vi "0.初始化饼状图.vi"(8 "error in":errorcluster) -> (0 "error out":errorcluster, 3 "Module ID out":i32)   [LabVIEW 2020, in "PichartInterface.lvlib"]
uses:
  PichartInterface.lvlib
  <vilib>/DD/DDToolsVIPM/PieChartInterface/PieChart.lvlibp
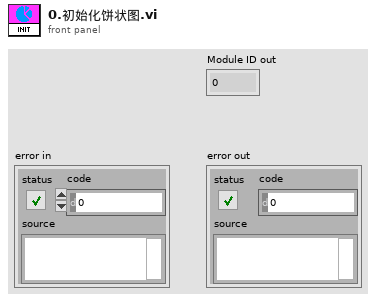
[diagram p1: front panel]
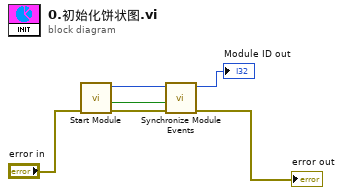
[diagram p0: block diagram]
diagram:
  n1 = call <vilib>:"Start Module.vi"("error in"="error in") -> ("error out"=w5:errorcluster, "Wait for Event Sync?"=w4:bool, "Module ID"=w6:i32)  [unwired: 7 in, 1 out]
  n2 = call <vilib>:"Synchronize Module Events.vi"("error in"=w5, "Wait for Event Sync?"=w4, "Module ID in"=w6) -> ("error out"=→"error out":errorcluster, "Module ID out"=→"Module ID out":i32)  [unwired: 7 in]
